vi "AIT 664 - Clear Database.vi"(8 "error in (no error)":errorcluster, 11 "Node Ptr":u64 format="%.0x") -> (0 "error out":errorcluster)   [LabVIEW 2013, in "AIT 664 Custom Device.lvlib"]
doc: "Clears the Veristand 664 configuration for a given card. Does not remove the card."
uses:
  AIT 664 Custom Device.lvlib
  Controls and Global/Global.vi
  <vilib>/NI Veristand/Custom Device API/Set Item Property (String).vi
  <vilib>/NI Veristand/Custom Device API/Custom Device API.lvlib
  <vilib>/NI Veristand/Custom Device Tools/Custom Device Utility Library/Custom Device Utility Library.lvlib
panel:
  in  "Tag":string
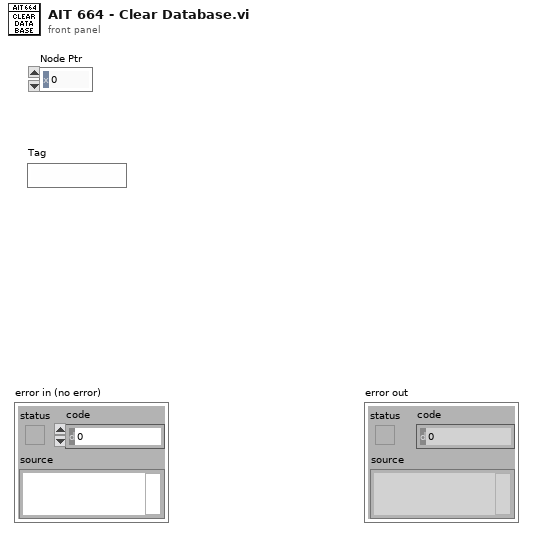
[diagram p1: front panel]
types:
  T1 = typedef "Custom Device API.lvlib/Custom Device Item Ref.ctl" = u64
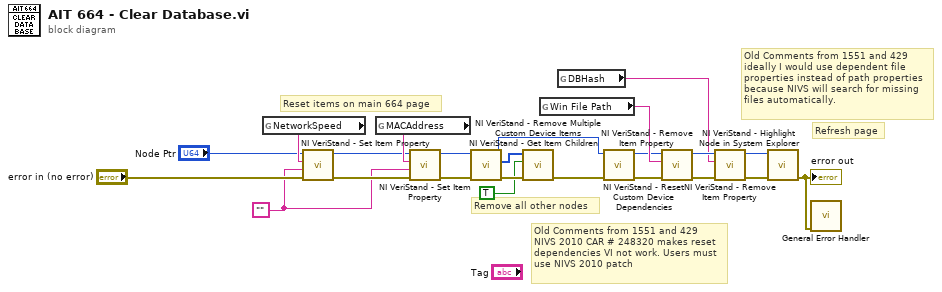
[diagram p0: block diagram]
diagram:
  w3 = ""
  # "Remove all other nodes"
  # "Reset items on main 664 page"
  # "Old Comments from 1551 and 429\nideally I would use dependent file properties instead of path properties because NIVS will search for missing files automatically."
  # "Old Comments from 1551 and 429\nNIVS 2010 CAR # 248320 makes reset dependencies VI not work. Users must use NIVS 2010 patch"
  # "Refresh page"
  n1 = global read "Global.vi" "NetworkSpeed"() -> (w6:string)
  n2 = call-poly <vilib>:"NI VeriStand - Set Item Property.vi"("error in (no error)"="error in (no error)", "Value"=w3, "Property Name"=w6, "Item Ref in"="Node Ptr") -> ("error out"=w7:errorcluster, "Item Ref out"=w8:T1)  [unwired: 5 in, 1 out]
  n3 = global read "Global.vi" "MACAddress"() -> (w9:string)
  n4 = call-poly <vilib>:"NI VeriStand - Set Item Property.vi"("error in (no error)"=w7, "Value"=w3, "Property Name"=w9, "Item Ref in"=w8) -> ("error out"=w5:errorcluster, "Item Ref out"=w1:T1)  [unwired: 5 in, 1 out]
  n5 = call <vilib>:"NI VeriStand - Get Item Children.vi"("error in (no error)"=w5, "Item Ref in"=w1) -> ("error out"=w23:errorcluster, "Child Refs"=w18:T1[], "Item Ref out"=w10:T1)  [unwired: 6 in, 1 out]
  n6 = call <vilib>:"NI VeriStand - Remove Multiple Custom Device Items.vi"("error in (no error)"=w23, "Force Delete (F)"=TRUE, "Item Refs in"=w18) -> ("error out"=w11:errorcluster)  [unwired: 7 in, 1 out]
  n7 = global read "Global.vi" "Win File Path"() -> (w20:string)
  n8 = global read "Global.vi" "DBHash"() -> (w12:string)
  n9 = call <vilib>:"NI VeriStand - Reset Custom Device Dependencies.vi"("error in (no error)"=w11, "Device Ref in"=w10) -> ("error out"=w21:errorcluster, "Device Ref out"=w19:T1)  [unwired: 8 in]
  n10 = call <vilib>:"NI VeriStand - Remove Item Property.vi"("error in (no error)"=w21, "Property Name"=w20, "Item Ref in"=w19) -> ("error out"=w16:errorcluster, "Item Ref out"=w15:T1)  [unwired: 6 in, 1 out]
  n11 = call <vilib>:"NI VeriStand - Remove Item Property.vi"("error in (no error)"=w16, "Property Name"=w12, "Item Ref in"=w15) -> ("error out"=w14:errorcluster, "Item Ref out"=w13:T1)  [unwired: 6 in, 1 out]
  n12 = call <vilib>:"NI VeriStand - Highlight Node in System Explorer.vi"("error in (no error)"=w14, "Item Ref in"=w13) -> ("error out"=w17:errorcluster)  [unwired: 8 in, 1 out]
  "error out" <- w17
  n13 = call <vilib>:"General Error Handler.vi"("error in (no error)"=w17) -> ()  [unwired: 10 in, 5 out]
